vi "SetExplicitMessage.vi"(6 "value":i32, 8 "error in (no error)":errorcluster, 10 "Motor Controller Parameter":T1, 11 ".NET Refnum in":refnum<k24>) -> (0 "error out":errorcluster, 1 "GetAttributeSingle":u8[](array[numeric]), 2 "size":i32, 3 ".NET Refnum out":refnum<k24>, 4 "Return Data (U32)":u32)   [LabVIEW 2022 SP3, in "Motor Controller.lvclass"]
uses:
  Motor Controller.lvclass
  C:/projects/Digilens_IPLC2/Classes/Motor Controller/EEIP.dll
  EEIP.dll
  Typedefs/Motor Controller Parameter-Set.ctl
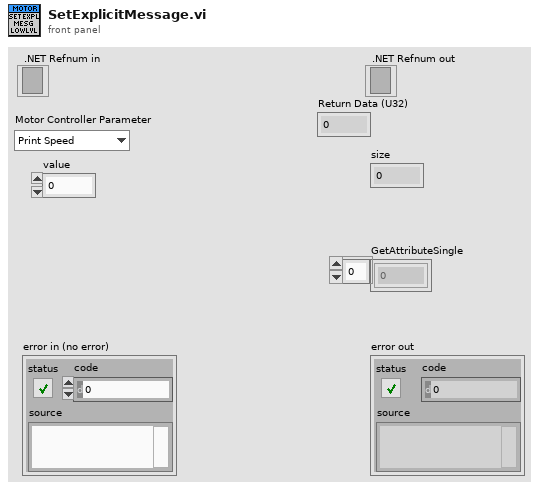
[diagram p1: front panel]
types:
  T1 = typedef "Motor Controller.lvclass/Motor Controller Parameter-Set.ctl" = enum16{"Print Speed", "Jog Speed", "PR Path", "Enable Servo", "Disable Servo", "Move Stage to Under PH1", "Move Stage to Under PH2", "Move Stage to Under PH3", "Move Stage to Under PH4", "Move Stage to Under PH5", "Move Stage to Under PH6", "Home Stage", "Return Stage to 0", "Print Stage", "Write Speed", "Write Index", "Stop Stage"}
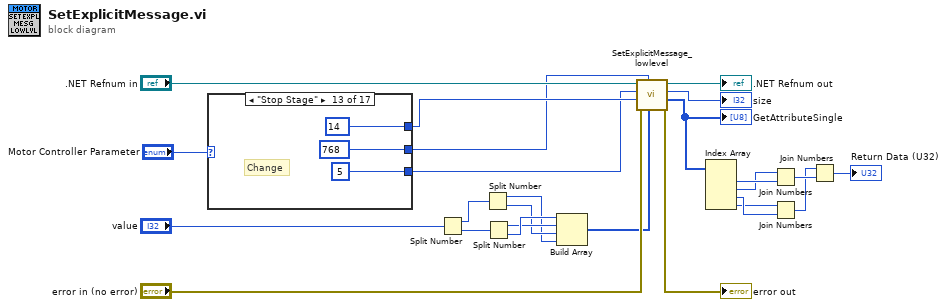
[diagram p0: block diagram]
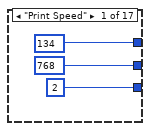
[diagram p2: hidden frame]
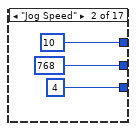
[diagram p3: hidden frame]
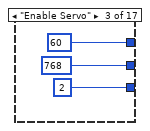
[diagram p4: hidden frame]
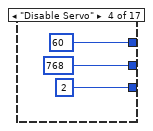
[diagram p5: hidden frame]
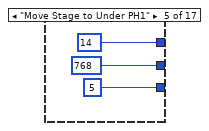
[diagram p6: hidden frame]
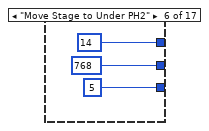
[diagram p7: hidden frame]
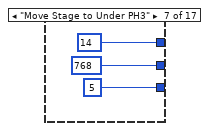
[diagram p8: hidden frame]
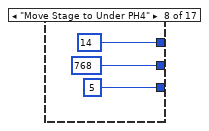
[diagram p9: hidden frame]
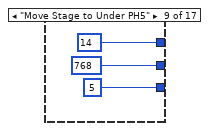
[diagram p10: hidden frame]
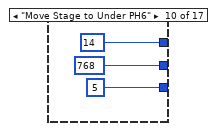
[diagram p11: hidden frame]
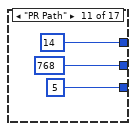
[diagram p12: hidden frame]
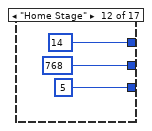
[diagram p13: hidden frame]
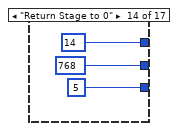
[diagram p14: hidden frame]
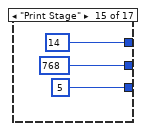
[diagram p15: hidden frame]
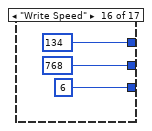
[diagram p16: hidden frame]
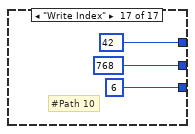
[diagram p17: hidden frame]
diagram:
  n1 = case shown="\"Stop Stage\"" "Motor Controller Parameter" {
    tunnel: [134 ("Attribute") 10 ("Attribute") 60 ("Attribute") 60 ("Attribute") 14 ("Attribute") 14 ("Attribute") 14 ("Attribute") 14 ("Attribute") 14 ("Attribute") 14 ("Attribute") 14 ("Attribute") 14 ("Attribute") 14 ("Attribute") 14 ("Attribute") 14 ("Attribute") 134 ("Attribute") 42 ("Attribute")] -> w19
    tunnel: [768 ("Class") 768 ("Class") 768 ("Class") 768 ("Class") 768 ("Class") 768 ("Class") 768 ("Class") 768 ("Class") 768 ("Class") 768 ("Class") 768 ("Class") 768 ("Class") 768 ("Class") 768 ("Class") 768 ("Class") 768 ("Class") 768 ("Class")] -> w18
    tunnel: [u32 2 ("assembly instance ID") u32 4 ("assembly instance ID") u32 2 ("assembly instance ID") u32 2 ("assembly instance ID") u32 5 ("assembly instance ID") u32 5 ("assembly instance ID") u32 5 ("assembly instance ID") u32 5 ("assembly instance ID") u32 5 ("assembly instance ID") u32 5 ("assembly instance ID") u32 5 ("assembly instance ID") u32 5 ("assembly instance ID") u32 5 ("assembly instance ID") u32 5 ("assembly instance ID") u32 5 ("assembly instance ID") u32 6 ("assembly instance ID") u32 6 ("assembly instance ID")] -> w17
    frame "Print Speed" {
    }
    frame "Jog Speed" {
    }
    frame "Enable Servo" {
    }
    frame "Disable Servo" {
    }
    frame "Move Stage to Under PH1" {
    }
    frame "Move Stage to Under PH2" {
    }
    frame "Move Stage to Under PH3" {
    }
    frame "Move Stage to Under PH4" {
    }
    frame "Move Stage to Under PH5" {
    }
    frame "Move Stage to Under PH6" {
    }
    frame "PR Path" {
    }
    frame "Home Stage" {
    }
    frame "Stop Stage" {
      # "Change"
    }
    frame "Return Stage to 0" {
    }
    frame "Print Stage" {
    }
    frame "Write Speed" {
    }
    frame "Write Index" {
      # "#Path 10"
    }
  }
  n2 = Split Number(x="value") -> (hi(x)=w15:u16, lo(x)=w16:u16)
  n3 = Split Number(x=w15) -> (hi(x)=w11:u8, lo(x)=w12:u8)
  n4 = Split Number(x=w16) -> (hi(x)=w13:u8, lo(x)=w14:u8)
  n5 = Build Array(w14, w13, w12, w11) -> (w9:u8[])
  n6 = call "SetExplicitMessage_lowlevel.vi"("value"=w9, "Class"=w18, "error in (no error)"="error in (no error)", "Attribute"=w19, "assembly instance ID"=w17, ".NET Refnum in"=".NET Refnum in") -> ("error out"=→"error out":errorcluster, "SetAttributeSingle"=w1:u8[], "Numeric"=→"size":i32, ".NET Refnum out"=→".NET Refnum out":refnum<k24>)  [unwired: 2 in]
  "GetAttributeSingle" <- w1
  n7 = Index Array(array=w1) -> (element #1=w8:u8, element #2=w7:u8, element #3=w6:u8, element #4=w5:u8)  [unwired: 4 in]
  n8 = Join Numbers(hi=w7, lo=w8) -> ((hi.lo)=w4:u16)
  n9 = Join Numbers(hi=w5, lo=w6) -> ((hi.lo)=w3:u16)
  n10 = Join Numbers(hi=w3, lo=w4) -> ((hi.lo)=→"Return Data (U32)":u32)
